vi "AlazarAcqPrep - ATS-SDK.vi"(0 "Handle":u32, 1 "Digitizer Settings":T1={"Digitizer delay (us) "=0.0, "rf points per line"=2048, "lines per plane"=128, "Samp Rate (Hz)"=100000000.0, "Additional dig delay (us)"=0.0, "Voltage Scale"=0.4, "Pre-Looks"=0, "Offset delay (us)"=0.0, "bits A/D"=8, "Avg Num"=1, "DigTimeOut"=5.0, "Rel Dig Delay"=0.0, "Dig Ch"=0, "LeCroyCluster"={"LeCroy Channels"=[TRUE, FALSE, FALSE, FALSE], "LC read pt offset"=0.0, "Sweep Avg"=FALSE}, "Main Digitizer"=enum."NI Digitizer", "Dig Config"=enum."Single channel", "Digitizer ID Cluster"={"Acqiris/Alazar/SP ID"=[], "NI Instr Handles"=[], "LeCroy VISA"="", "GaGe Handle"={"Handle"=0, "Sample size"=0, "Resolution"=0, "Offset"=0, "Channels"=0, "Boards"=0}, "ATS Ref"="ATS9350", "Acqiris Address"=["PCI::INSTR0"], "ADQRef"=refnum, "adq_cu_ptr"=refnum}, "Trigger Settings"={"Trig Source"=1, "Trig Coupling"=0, "Trig Slope"=0, "Level (mV)"=1500.0}, "Bulk Acq"=FALSE, "Bulk Start Indexes"=[], "Data Ref RF"=refnum, "NI ID/Channel"=[], "Total Dig CH"=1, "Xtra Ann Trig delay (us)"=10.0, "Fix Z Delay?"=FALSE, "One Way Transmission?"=FALSE, "Data Ref Log"=refnum} {"Trigger Settings"."Trig Slope" items=["Positive", "Negative"]; "Trigger Settings"."Level (mV)" format="%.2f"; "Trigger Settings"."Trig Coupling" items=["DC 1 MOhm", "AC 1 MOhm", "DC 50 Ohm", "AC 50 Ohm"]; "Trigger Settings"."Trig Source" items=["Chan 1", "External"]; "Rel Dig Delay" format="%.2f"; "DigTimeOut" format="%.2f"; "Avg Num" min=1; "Offset delay (us)" format="%.2f"; "Additional dig delay (us)" format="%.2f"; "Digitizer delay (us)" format="%.2f"}, 2 "LimitBuffers?":bool, 3 "Enable Trigger Enable":bool, 5 "Channel":u32(ring)=1 items=["A"=1, "B"=2, "A + B"=3, "C"=4, "A + C"=5, "A + B"=6, "D"=8, "A + D"=9, "B + D"=10, "C + D"=12, "A + B + C + D"=15], 7 "BuffCount":i32=4, 9 "rf points per line":i32, 11 "error in (no error)":errorcluster, 12 "rf lines per buffer":i32) -> (4 "Handle Out":u32, 6 "AlazarCluster":T5, 10 "Return Code":u32, 15 "error out":errorcluster)   [LabVIEW 2022 SP3]
uses:
  -DigitizerRoutines/DigitizerSettings.ctl
  -DigitizerRoutines/Digitizer.ctl
  -DigitizerRoutines/DigConfig.ctl
  -DigitizerRoutines/DigitizerID.ctl
  C:/Windows/System32/ADQAPI_dotNet_helper.dll
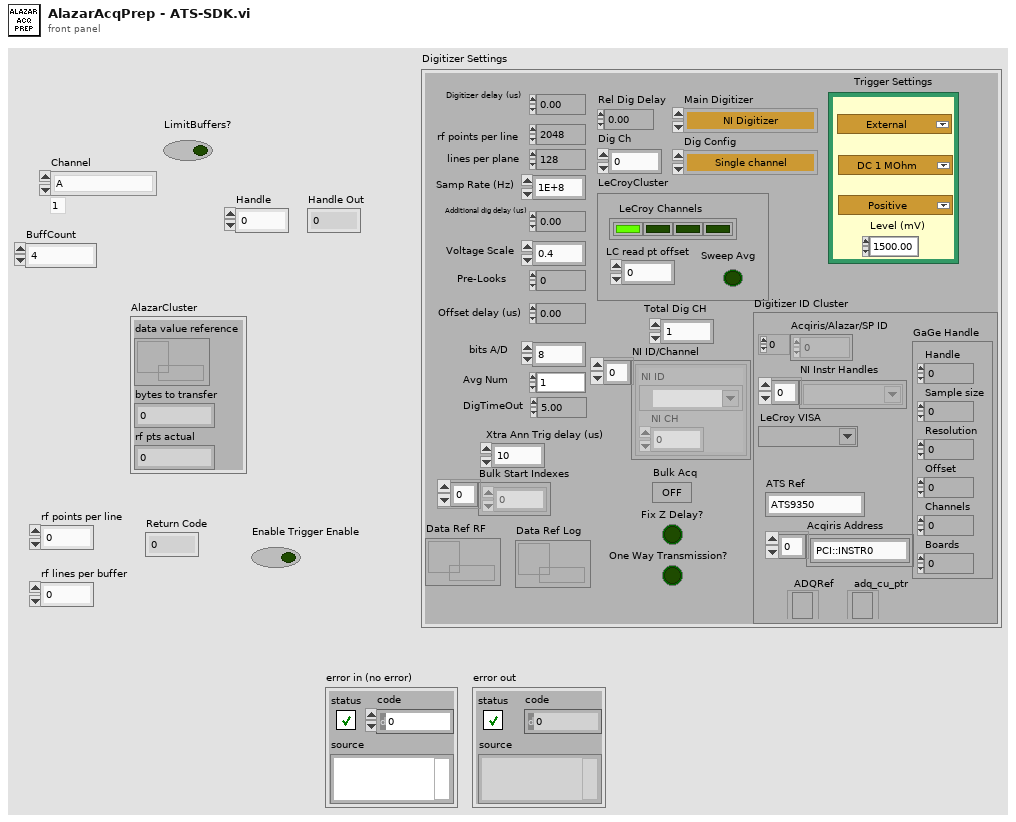
[diagram p1: front panel]
types:
  T1 = typedef "DigitizerSettings.ctl" = cluster{"Digitizer delay (us) ":dbl, "rf points per line":i32, "lines per plane":i32, "Samp Rate (Hz)":dbl, "Additional dig delay (us)":dbl, "Voltage Scale":dbl, "Pre-Looks":i32, "Offset delay (us)":dbl, "bits A/D":i8, "Avg Num":i32, "DigTimeOut":sgl, "Rel Dig Delay":sgl, "Dig Ch":i32, "LeCroyCluster":cluster{"LeCroy Channels":bool[], "LC read pt offset":dbl, "Sweep Avg":bool}, "Main Digitizer":T2, "Dig Config":T3, "Digitizer ID Cluster":T4, "Trigger Settings":cluster{"Trig Source":u16, "Trig Coupling":u16, "Trig Slope":u16, "Level (mV)":dbl}, "Bulk Acq":bool, "Bulk Start Indexes":i32[], "Data Ref RF":refnum<data-value>, "NI ID/Channel":cluster{"NI ID":refnum<k15>, "NI CH":i32}[], "Total Dig CH":i32, "Xtra Ann Trig delay (us)":dbl, "Fix Z Delay?":bool, "One Way Transmission?":bool, "Data Ref Log":refnum<data-value>}
  T2 = typedef "Digitizer.ctl" = enum16{"Acqiris Digitizer", "NI Digitizer", "LeCroy", "GaGe", "AlazarTech", "No Digitizer", "Teledyne"}
  T3 = typedef "DigConfig.ctl" = enum16{"Single channel", "2 Chans w/ 2 Acqiris", "2 Chans w/ 1 Acqiris", "5-CH Pulser New", "5-CH pulser w/ ann array", "5-pass style ann array", "Empty"}
  T4 = typedef "DigitizerID.ctl" = cluster{"Acqiris/Alazar/SP ID":u32[], "NI Instr Handles":refnum<k15>[], "LeCroy VISA":refnum<visa-resource-name>, "GaGe Handle":cluster{"Handle":u32, "Sample size":u32, "Resolution":i32, "Offset":i32, "Channels":u32, "Boards":u32}, "ATS Ref":string, "Acqiris Address":string[], "ADQRef":refnum<k24>, "adq_cu_ptr":refnum<k24>}
  T5 = cluster{"data value reference":refnum<data-value>, "bytes to transfer":u32, "rf pts actual":u32}
  T6 = cluster{"data value reference":refnum<data-value>, "Samples Per Buffer":u32, "y":u32}
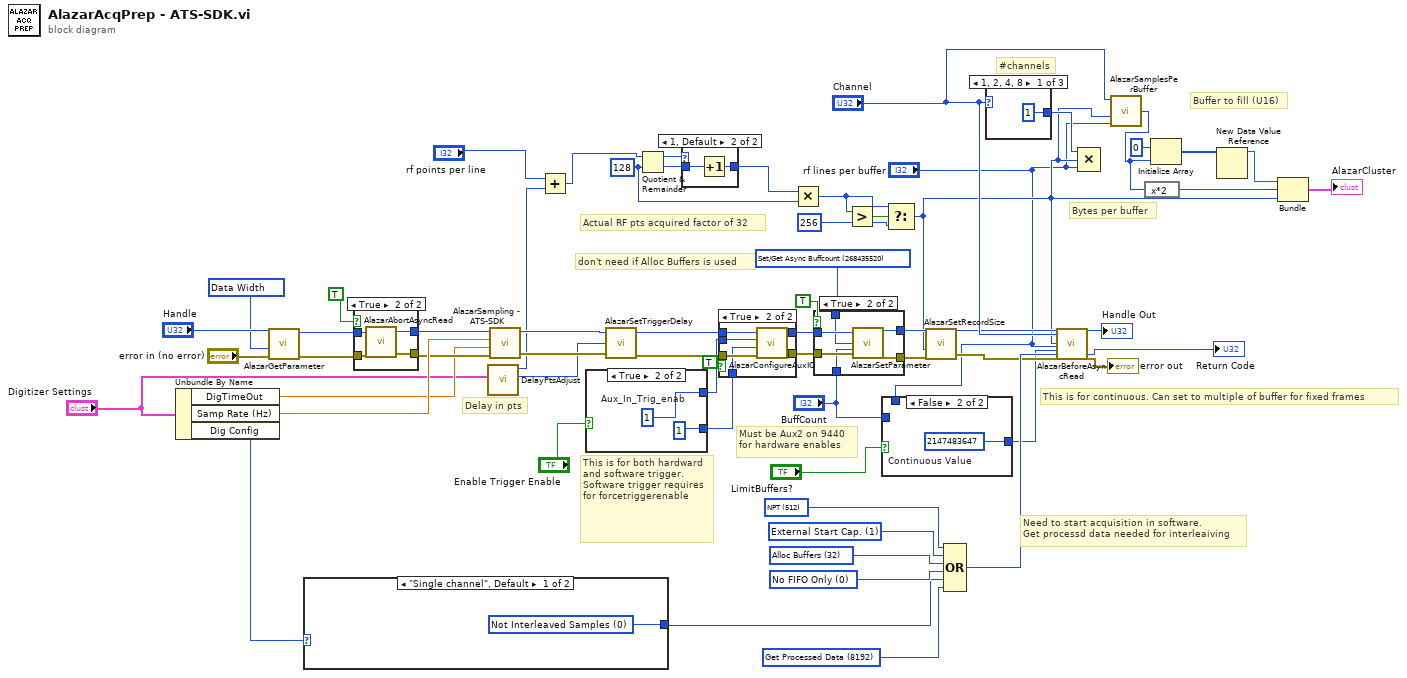
[diagram p0: block diagram]
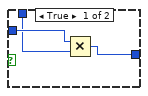
[diagram p3: hidden frame]
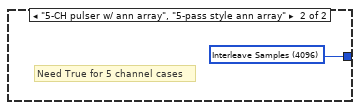
[diagram p5: hidden frame]
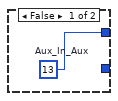
[diagram p6: hidden frame]
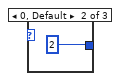
[diagram p9: hidden frame]
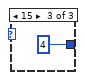
[diagram p10: hidden frame]
diagram:
  w19 = u32 256 ("y")
  w35 = u32 8192 items=["No Get Processed Data"=32, "Get Processed Data"=8192]
  w39 = u32 0 items=["No FIFO Only"=0, "FIFO Only"=2048]
  w36 = u32 32 items=["Alloc Buffers"=32]
  w37 = u32 1 items=["Internal Start Cap.", "External Start Cap."]
  w38 = u32 512 items=["Traditional"=0, "NPT"=512, "Continuous"=256, "Triggered Streaming"=1024]
  w40 = u32 268435465 items=["Data Width"=268435465, "Set/Get Async BuffSize"=268435513, "Set/Get Async Buffcount"=268435520, "Get Data Format"=268435522, "Get Samples Per Timestamp Clock"=268435524, "Get Records Captured"=268435525, "Get Async Buffers Pending"=268435536, "Get Async Buffers Pending Full"=268435537, "Get Async Buffers Pending Empty"=268435538, "ECC Mode"=268435528, "Get Aux Input Level"=268435529, "Get Channels Per Board"=268435568, "Pack Mode"=268435570, "Get FPGA Temperature"=268435584] ("Parameter")
  w45 = u32 268435520 items=["Set Single Chan."=268435523, "Data Width"=268435465, "Set/Get Async BuffSize"=268435513, "Set/Get Async Buffcount"=268435520, "Get Data Format"=268435522, "Get Samples Per Timestamp Clock"=268435524, "Get Records Captured"=268435525, "Get Async Buffers Pending"=268435536, "Get Async Buffers Pending Full"=268435537, "Get Async Buffers Pending Empty"=268435538, "ECC Mode"=268435528, "Get Aux Input Level"=268435529, "Get Channels Per Board"=268435568, "Pack Mode"=268435570, "Get FPGA Temperature"=268435584] ("Parameter")
  w59 = u32 128 ("y")
  # "don't need if Alloc Buffers is used"
  # "This is for continuous. Can set to multiple of buffer for fixed frames"
  # "Need to start acquisition in software.\nGet processd data needed for interleaiving"
  # "This is for both hardward and software trigger.\nSoftware trigger requires for forcetriggerenable"
  # "Must be Aux2 on 9440\nfor hardware enables"
  # "Actual RF pts acquired factor of 32"
  # "Buffer to fill (U16)"
  # "Bytes per buffer"
  # "#channels"
  # "Delay in pts"
  n1 = Unbundle By Name("Digitizer Settings") -> ("DigTimeOut"=w29:sgl, "Samp Rate (Hz)"=w52:dbl, "Dig Config"=w17:T3)
  n2 = call "AlazarGetParameter.vi"("error in (no error)"="error in (no error)", "Parameter"=w40, "Handle"="Handle") -> ("error out"=w42:errorcluster, "Handle"=w41:u64)  [unwired: 1 in, 2 out]
  n3 = case shown="\"Single channel\", Default" w17 {
    tunnel: [w63 w64] -> w32
    frame "Single channel", Default {
      w63 = u32 0 items=["Not Interleaved Samples"=0, "Interleave Samples"=4096]
    }
    frame "5-CH pulser w/ ann array", "5-pass style ann array" {
      w64 = u32 4096 items=["Not Interleaved Samples"=0, "Interleave Samples"=4096]
      # "Need True for 5 channel cases"
    }
  }
  n4 = case shown="True" TRUE {
    tunnel: w41 -> [w66 w70]
    tunnel: [w66 w69] -> w51
    tunnel: [w65 w68] -> w50
    tunnel: w42 -> [w65 w67]
    frame False {
    }
    frame True {
      n5 = call "AlazarAbortAsyncRead.vi"("Handle"=w70, "error in (no error)"=w67) -> ("Handle"=w69:u64, "error out"=w68:errorcluster)  [unwired: 1 out]
    }
  }
  n6 = call "DelayPtsAdjust.vi"("Digitizer Settings"="Digitizer Settings") -> ("Actual Delay pts"=w11:u32, "PostDelayCorrection"=w10:u32)  [unwired: 9 in]
  n7 = call "AlazarSampling - ATS-SDK.vi"("error in (no error)"=w50, "Time Out (s)"=w29, "Sampling (Hz)"=w52, "Handle"=w51) -> ("error out"=w13:errorcluster, "Handle Out"=w16:u32)  [unwired: 5 in, 1 out]
  n8 = Add(x="rf points per line", y=w10) -> (x+y=w8:u32)
  n9 = case shown="True" "Enable Trigger Enable" {
    tunnel: [w71 w73] -> w48
    tunnel: [_ u32 1] -> w1
    frame False {
      w71 = u32 13  # Aux_In_Aux
    }
    frame True {
      w73 = u32 1  # Aux_In_Trig_enab
    }
  }
  n10 = call "AlazarSetTriggerDelay.vi"("error in (no error)"=w13, "Delay"=w11, "Handle"=w16) -> ("error out"=w14:errorcluster, "Handle"=w15:u64)  [unwired: 1 out]
  n11 = Quotient & Remainder(x=w8, y=w59) -> (x-y*floor(x/y)=w54:u32, floor(x/y)=w60:u32)
  n12 = case shown="1, Default" w54 {
    tunnel: [w74 w76] -> w26
    tunnel: w60 -> [w74 w75]
    frame 0 {
    }
    frame 1, Default {
      n13 = Increment(x=w75) -> (x+1=w76:u32)
    }
  }
  n14 = case shown="True" TRUE {
    tunnel: w48 -> [_ w84]
    tunnel: [w77 w83] -> w47
    tunnel: [w78 w82] -> w46
    tunnel: w15 -> [w77 w81]
    tunnel: w14 -> [w78 w80]
    tunnel: w1 -> [_ w79]
    frame False {
    }
    frame True {
      n15 = call "AlazarConfigureAuxIO.vi"("error in (no error)"=w80, "Parameter"=w79, "Mode"=w84, "Handle"=w81) -> ("error out"=w82:errorcluster, "Handle"=w83:u64)  [unwired: 1 out]
    }
  }
  n16 = Multiply(x=w26, y=w59) -> (x*y=w20:u32)
  n17 = case shown="True" TRUE {
    tunnel: w47 -> [w86 w92]
    tunnel: w46 -> [w85 w91]
    tunnel: w45 -> [_ w90]
    tunnel: "BuffCount" -> [_ w89]
    tunnel: [w86 w88] -> w22
    tunnel: [w85 w87] -> w25
    frame False {
    }
    frame True {
      n18 = call "AlazarSetParameter.vi"("Handle"=w92, "Parameter"=w90, "Value"=w89, "error in (no error)"=w91) -> ("Handle"=w88:u64, "error out"=w87:errorcluster)  [unwired: 9 in, 1 out]
    }
  }
  n19 = Greater?(x=w20, y=w19) -> (0:w21:bool)
  n20 = case shown="False" "LimitBuffers?" {
    tunnel: [w94 w96] -> w7
    tunnel: "BuffCount" -> [w95 _]
    tunnel: "rf lines per buffer" -> [w93 _]
    frame True {
      n21 = Multiply(x=w95, y=w93) -> (x*y=w94:i32)
    }
    frame False {
      w96 = u32 2147483647  # Continuous Value
    }
  }
  n22 = Select(t=w20, s=w21, f=w19) -> (s? t:f=w18:u32)
  n23 = call "AlazarSetRecordSize.vi"("error in (no error)"=w25, "Post-trigger Samples"=w18, "Handle"=w22) -> ("error out"=w24:errorcluster, "Handle"=w23:u64)  [unwired: 1 in, 1 out]
  n24 = Compound Arithmetic op=OR(w38, w37, w36, w39, w32, w35) -> (w33:u32)
  n25 = case shown="1, 2, 4, 8" "Channel" {
    tunnel: [u32 1 ("value") u32 2 ("value") u32 4 ("value")] -> w58
    frame 1, 2, 4, 8 {
    }
    frame 0, Default {
    }
    frame 15 {
    }
  }
  n26 = call "AlazarBeforeAsyncRead.vi"("Handle"=w23, "Channel Select"="Channel", "Transfer Length"=w18, "Records Per Buffer"="rf lines per buffer", "Records Per Acquisition"=w7, "Flags"=w33, "error in (no error)"=w24) -> ("Handle"=→"Handle Out":u64, "Return Code"=→"Return Code":u32, "error out"=→"error out":errorcluster)  [unwired: 18 in]
  n27 = Compound Arithmetic op=MULTIPLY(w58, w18, "rf lines per buffer") -> ()  [unwired: 1 out]
  n28 = call "AlazarSamplesPerBuffer.vi"("Records Per Buffer"="rf lines per buffer", "Samples Per Record"=w18, "Channel Mask"="Channel") -> ("Samples Per Buffer"=w28:u32)  [unwired: 1 in]
  n29 = expression code="x*2"(w28) -> (w62:u32)
  n30 = Initialize Array(u16 0, w28) -> (w57:u16[])
  n31 = New Data Value Reference(data value=w57) -> (data value reference=w56:refnum<data-value>)  [unwired: 1 in, 1 out]
  n32 = Bundle("data value reference"=w56, "Samples Per Buffer"=w62, "y"=w18) -> (→"AlazarCluster":T6)  [unwired: 1 in]
